vi "CSM - Register Status Change.vi"(0 "CSM Name":string, 5 "Source CSM Name (* as Default)":string="*", 7 "Status":string, 9 "Response Message (If \"\", Same as Source Message)":string, 11 "Error In":errorcluster caption="error in (no error)") -> (4 "CSM Name (Dup)":string, 15 "error out":errorcluster)   [LabVIEW 2017, in "Communicable State Machine.lvlib"]
doc: "This VI is obsolete. Please use `CSM - Register Broadcast.vi`\n\n## CSM - Register Broadcast.vi\nRegisters to receive notifications of changes triggered by other CSM modules. If <b>API</b> is not wired or the input is empty, the trigger name will be used as the response message. The trigger name can be the broadcast name of the source module or the state name of the source module.\n\nIn Worker Mode and Chain of Responsibility Mode, the input node name is automatically parsed as the module name because CSM implements registrations on a per-module basis.\n\n<b>Reference Example</b>: `2. Caller is CSM Scenario\\CSM Example - Caller is a CSM.vi`.\n\n> - Ref: CSM Registration\n> - Ref: CSM Registration Location\n> - Ref: CSM Broadcast Priority\n\n-- <b>Controls</b> --\n- <b>CSM Name</b>: CSM module name.\n- <b>Source CSM Name (* as Default)</b>: The CSM module generating the status. You can use `*` to represent all modules generating the same status.\n- <b>Trigger</b>: Trigger string.\n- <b>API (if \"\", same as Trigger)</b>: Upon registration, this message will be received if the trigger changes.\n- <b>Priority (No Change)</b>: Broadcast priority after registration.\n\n-- <b>Indicators</b> --\n- <b>CSM Name (Dup)</b>: A copy of the input CSM module name."
uses:
  Communicable State Machine.lvlib
  CSM - Broadcast Message Type.ctl
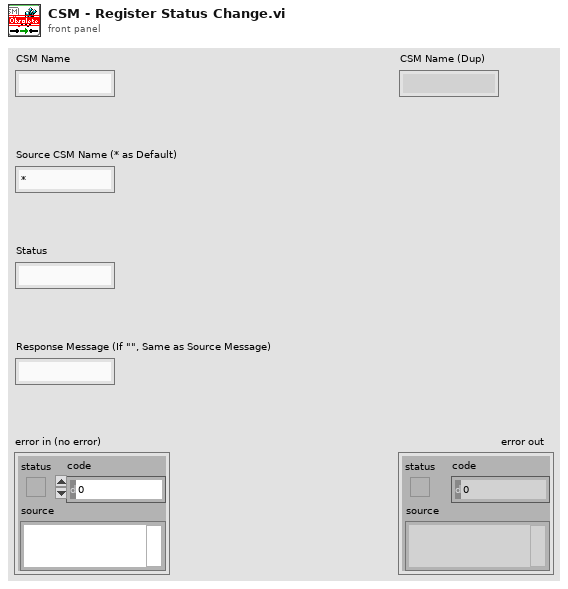
[diagram p1: front panel]
types:
  T1 = typedef "Communicable State Machine.lvlib/CSM - Broadcast Message Type.ctl" = enum16{"<Null>", "Status", "Interrupt"}
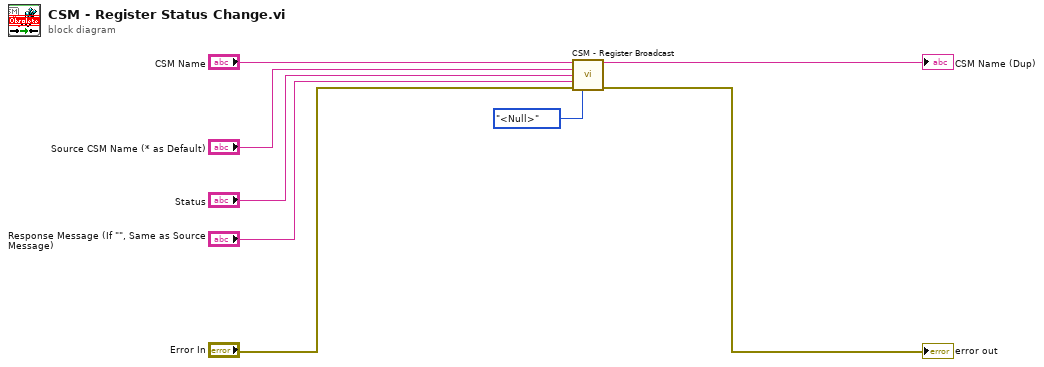
[diagram p0: block diagram]
diagram:
  n1 = call "CSM - Register Broadcast.vi"("CSM Name(Empty for Broadcast Event)"="CSM Name", "Source CSM Name (* as Default)"="Source CSM Name (* as Default)", "Trigger"="Status", "API (If \"\", Same as Trigger)"="Response Message (If \"\", Same as Source Message)", "Error In"="Error In", "Priority (No Change)"=CSM_-_Broadcast_Message_Type."<Null>" ("Priority(No Change)")) -> ("CSM Name (Dup)"=→"CSM Name (Dup)":string, "error out"=→"error out":errorcluster)  [unwired: 8 in]
